vi "New JSON Array (Empty).vi"(8 "error in (no error)":errorcluster) -> (0 "error out":errorcluster, 3 "JSON Array out":refnum<class "JSON Helper.lvclass">)   [LabVIEW 2016, in "JSON Helper.lvclass"]
doc: "Creates a new empty JSON Array"
uses:
  JSON Helper/JSON Helper.lvclass
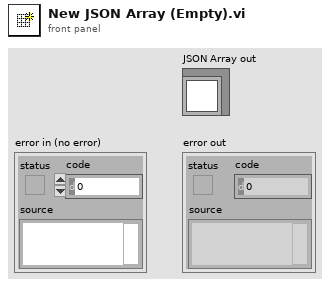
[diagram p1: front panel]
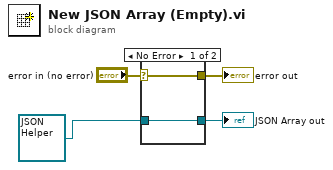
[diagram p0: block diagram]
diagram:
  n1 = case shown="No Error" "error in (no error)" {
    selector: "error in (no error)" -> [w5 w8]
    tunnel: [w5 w8] -> w3
    tunnel: [w6 w7] -> w2
    tunnel: refnum<class "JSON Helper.lvclass"> refnum ("JSON out") -> [w6 w7]
    frame No Error {
    }
    frame Error {
    }
  }
  "error out" <- w3
  "JSON Array out" <- w2
